vi "Software Initialisation.vi"(8 "error in (no error)":errorcluster, 11 "UI elements cluster":T2) -> (0 "Error Out":errorcluster, 2 "Event Registration Refnum":refnum<event-registration>, 3 "Message Queues out":T1)   [LabVIEW 2020]
uses:
  Typedefs/Top level VI states.ctl
  Typedefs/UI ctrl refs cluster.ctl
  Typedefs/Laser control knob.ctl
  Typedefs/Frame Size.ctl
  Typedefs/Plane Mode.ctl
  Typedefs/PMT control knob.ctl
  Typedefs/XY Stage_Move.ctl
  Typedefs/test_fpga_control.ctl
  Acquisition/Typedefs/Ref DAQ Param.ctl
  User Interface/Misc/Experiment Type.ctl
  User Interface/Misc/Biology Information.ctl
  User Interface/Queue/Message Queue/Typedefs/All Message Queues.ctl
  User Interface/Queue/Message Queue/Typedefs/Message Cluster.ctl
  Typedefs/Logging queue element.ctl
  Typedefs/Imaging Protocols enum.ctl
  Typedefs/Acquired points count.ctl
  Error window positioning/Error window pos FGV states.ctl
  Typedefs/Save-Load enum.ctl
  Global Variables/gl_UI Ctrl Refs.vi
  Global Variables/General Globals.vi
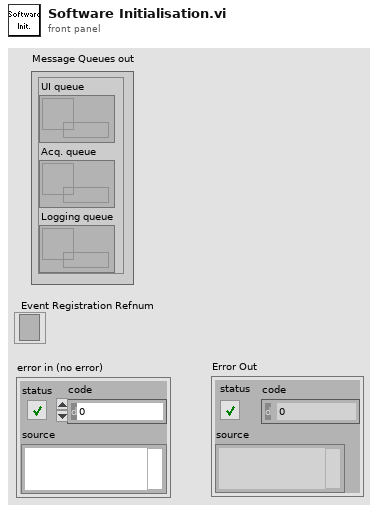
[diagram p1: front panel]
types:
  T1 = typedef "All Message Queues.ctl" = cluster{"UI queue":refnum<queue>, "Acq. queue":refnum<queue>, "Logging queue":refnum<queue>}
  T2 = typedef "UI ctrl refs cluster.ctl" = cluster{"Top level VI path":path, "Top level VI ref":refnum<vi>, "User menu ref":refnum<k9>, "Sub Panel control":refnum<vi>, "Imaging Param Tab":refnum<vi>, "Occurrence-Start drivers":refnum<k4>, "Occurrence-Speed logging initialised":refnum<k4>, "Occurrence-XYZ stage initialised":refnum<k4>, "Exit button":refnum<vi>, "Status ind":refnum<vi>, "Set as origin":refnum<vi>, "Speed Logging":refnum<vi>, "Time Lapse":refnum<vi>, "Live Imaging":refnum<vi>, "AOL Z Stack":refnum<vi>, "Motor Z Stack":refnum<vi>, "Funct Acq button":refnum<vi>, "Hard Shutter":refnum<vi>, "Virtual Shutter":refnum<vi>, "Laser Power":refnum<vi>, "AOL Mode":refnum<vi>, "Frame Size":refnum<vi>, "Field of View":refnum<vi>, "Dwell Time":refnum<vi>, "Zoom":refnum<vi>, "AOL Z":refnum<vi>, "Objective":refnum<vi>, "Axis":refnum<vi>, "Paths & Names":refnum<vi>, "Experiment folder path (ind.)":refnum<vi>, "Last State (Ind.)":refnum<vi>, "Averages":refnum<vi>, "Angle (degrees)":refnum<vi>, "X centre":refnum<vi>, "Y centre":refnum<vi>, "Plane Mode":refnum<vi>, "# Planes":refnum<vi>, "Z Start":refnum<vi>, "Z Stop":refnum<vi>, "Z Step":refnum<vi>, "PMT 1":refnum<vi>, "PMT 2":refnum<vi>, "Stage XYZ Position":refnum<vi>, "Pockels@Z Start":refnum<vi>, "Pockels@Z Stop":refnum<vi>, "Obtain Z Start":refnum<vi>, "Obtain Z Stop":refnum<vi>, "Live stim.trig.period":refnum<vi>, "Live stim.trig.enable":refnum<vi>, "Movement Correction":refnum<vi>, "Load Reference Image":refnum<vi>, "XY Stage Move":refnum<vi>, "MovCor Cluster":refnum<vi>, "RefDAQParam":refnum<vi>, "Funct. Acq. Pockels Modulation":refnum<vi>, "Ref Laser Power":refnum<vi>, "Enable Video Recording":refnum<vi>, "Video Record-Live Imaging":refnum<vi>, "Video Record-Funct acq":refnum<vi>, "Reference Source":refnum<vi>, "AOL Z-stack Chirps Ready (ind)":refnum<vi>, "Target time between mov.cor. ref triggers (ms)":refnum<vi>, "Funct. Acq. Ref frame save":refnum<vi>, "Tracking button":refnum<vi>, "Show ref plots window":refnum<vi>, "Center freq ind (nm)":refnum<vi>, "Pickup mode (ind)":refnum<vi>, "Logging queue (ind)":refnum<vi>, "Back aperture power (ind.)":refnum<vi>, "Power after objective (ind.)":refnum<vi>, "Switch user":refnum<vi>, "Ls1 Conn. Status":refnum<vi>, "Ls1Tuning Status":refnum<vi>, "Ls1 Faults":refnum<vi>, "Ls1 Connection":refnum<vi>, "Ls1 Mode":refnum<vi>, "Ls1 POWER [mW]":refnum<vi>, "Ls1Shutter":refnum<vi>, "Ls1 Wavelength":refnum<vi>, "Ls1 Note":refnum<vi>, "Ls1 Confirm Wav":refnum<vi>, "Ls1 PreChrp Prism1":refnum<vi>, "Ls1 PreChrp Prism2":refnum<vi>, "Ls1 wav top Ind":refnum<vi>, "Ls1 power top Ind":refnum<vi>, "Ls1 Pump peak Hold":refnum<vi>, "Ls1 Status Ind":refnum<vi>, "Ls1 wav cancel":refnum<vi>, "Experiment Type":refnum<vi>, "Biology Information":refnum<vi>, "Camera recording status":refnum<vi>, "Optimise Obj. Pos.":refnum<vi>}
  T3 = typedef "Save-Load enum.ctl" = enum16{"Save to file", "Load from file", "Compare from file", "Save Backup"}
  T4 = enum32{"Invalid", "Standard", "Closed", "Hidden", "Minimized", "Maximized"}
  T5 = typedef "Error window pos FGV states.ctl" = enum16{"Read", "Window closed", "Window opened", "Reset"}
  T6 = enum16{"Obtain queue", "Call window", "Call & send signal", "Release queue"}
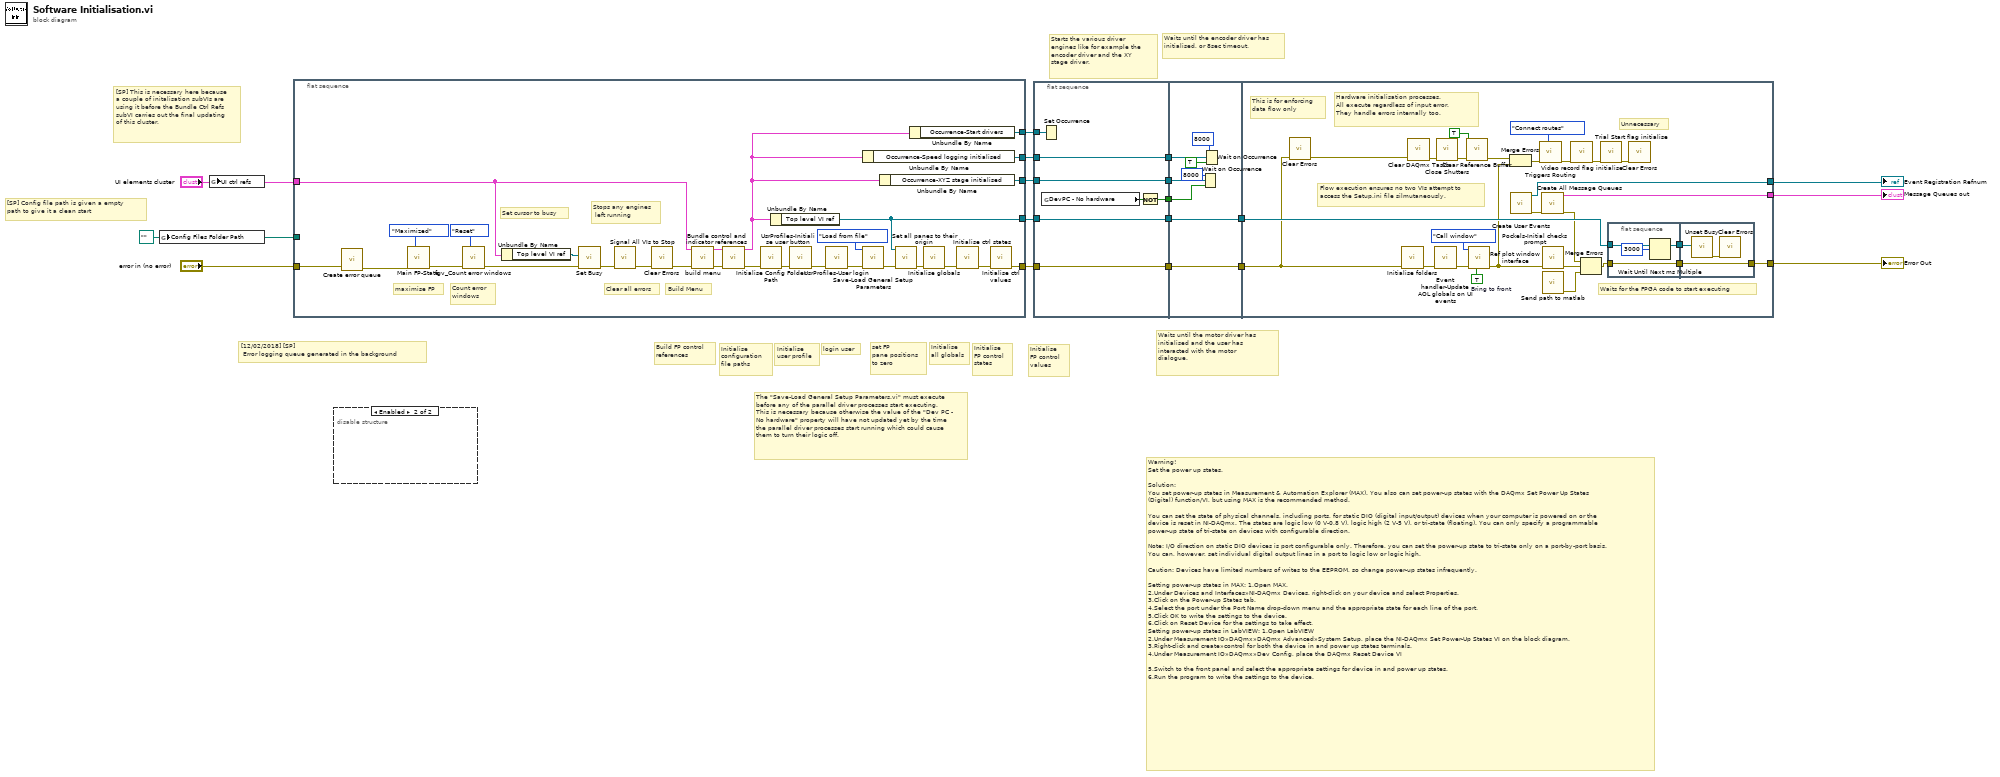
[diagram p0: block diagram]
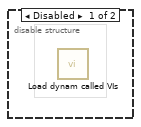
[diagram p2: hidden frame]
diagram:
  w13 = path "" ("Config Files Folder Path")
  # "[12/02/2018] [SP]\n Error logging queue generated in the background"
  # "[SP] Config file path is given a empty \npath to give it a clean start"
  # "Initialise \nFP control\nvalues"
  # "Initialise \nFP control\nstates"
  # "Initialise \nall globals"
  # "set FP \npane positions\nto zero"
  # "login user"
  # "Initialise \nuser profile"
  # "Initialise \nconfiguration\nfile paths"
  # "Build FP control\nreferences"
  # "Waits until the motor driver has initialised and the user has interacted with the motor dialogue."
  # "Starts the various driver engines like for example the encoder driver and the XY stage driver."
  # "Waits until the encoder driver has initialised, or 8sec timeout."
  # "The \"Save-Load General Setup Parameters.vi\" must execute before any of the parallel driver processes start executing. This is necessary because otherwise the value of the \"Dev PC - No hardware\" property will have not updated yet by the time the parallel driver processes start running which could cause them to turn their logic off."
  # "[SP] This is necessary here because a couple of initalisation subVIs are using it before the Bundle Ctrl Refs subVI carries out the final updating of this cluster."
  # "Warning!\nSet the power up states.\n\nSolution: \nYou set power-up states in Measurement & Automation Explorer (MAX). You also can set power-up states with the DAQmx Set Power Up States (Digital) function/VI, but using MAX is the recommended method. \n\nYou can set the state of physical channels, including ports, for static DIO (digital input/output) devices when your computer is powered on or the device is reset in NI-DAQmx. The states are logic low (0 V-0.8 V), logic high (2 V-5 V), or tri-state (floating). You can only specify a programmable power-up state of tri-state on devices with configurable direction. \n\nNote: I/O direction on static DIO devices is port configurable only. Therefore, you can set the power-up state to tri-state only on a port-by-port basis. You can, however, set individual digital output lines in a port to logic low or logic high.\n\nCaution: Devices have limited numbers of writes to the EEPROM, so change power-up states infrequently.\n\nSetting power-up states in MAX: 1.Open MAX.\n2.Under Devices and Interfaces»NI-DAQmx Devices, right-click on your device and select Properties.\n3.Click on the Power-up States tab.\n4.Select the port under the Port Name drop-down menu and the appropriate state for each line of the port.\n5.Click OK to write the settings to the device.\n6.Click on Reset Device for the settings to take effect.\nSetting power-up states in LabVIEW: 1.Open LabVIEW\n2.Under Measurement IO»DAQmx»DAQmx Advanced»System Setup, place the NI-DAQmx Set Power-Up States VI on the block diagram.\n3.Right-click and create»control for both the device in and power up states terminals.\n4.Under Measurement IO»DAQmx»Dev Config, place the DAQmx Reset Device VI \n\n5.Switch to the front panel and select the appropriate settings for device in and power up states.\n6.Run the program to write the settings to the device."
  n1 = global write "General Globals.vi" "Config Files Folder Path"(w13) -> ()
  n2 = global write "gl_UI Ctrl Refs.vi" "UI ctrl refs"("UI elements cluster") -> ()
  n3 = flat-sequence {
    tunnel: "error in (no error)" -> [w21]
    tunnel: "UI elements cluster" -> [w38]
    tunnel: [w34] -> w8
    tunnel: [w33] -> w9
    tunnel: [w32] -> w10
    tunnel: [w31] -> w11
    tunnel: w13 -> [_]
    tunnel: [w30] -> w12
    frame #0 {
      # "Build Menu"
      # "Clear all errors"
      # "Stops any engines\n left running"
      # "Set cursor to busy"
      # "maximise FP"
      # "Count error\nwindows"
      n4 = call "Create error queue.vi"("Error in"=w21) -> ("Error out"=w20:errorcluster)  [unwired: 10 in]
      n5 = call "Main FP-State.vi"("error in (no error)"=w20, "Front Panel Window:State"=T4."Maximized") -> ("error out"=w39:errorcluster)  [unwired: 9 in]
      n6 = call "fgv_Count error windows.vi"("error in (no error)"=w39, "Function"=Error_window_pos_FGV_states."Reset") -> ("error out"=w41:errorcluster)  [unwired: 7 in, 2 out]
      n7 = Unbundle By Name(w38) -> ("Top level VI ref"=w44:refnum<vi>)
      n8 = call <vilib>:"Set Busy.vi"("error in (no error)"=w41, "VI reference (current VI)"=w44) -> ("error out"=w46:errorcluster)  [unwired: 8 in, 1 out]
      n9 = call "Signal All VIs to Stop.vi"("error in (no error)"=w46) -> ("error out"=w36:errorcluster)  [unwired: 10 in]
      n10 = call <vilib>:"Clear Errors.vi"("error in (no error)"=w36) -> ("error out"=w35:errorcluster)  [unwired: 5 in, 1 out]
      n11 = call "build menu.vi"("error in (no error)"=w35, "UI elements cluster"=w38) -> ("error out"=w45:errorcluster, "UI elements cluster"=w37:T2)  [unwired: 8 in]
      n12 = call "Bundle control and indicator references.vi"("error in"=w45, "UI elements cluster"=w37) -> ("error out"=w19:errorcluster, "UI elements cluster"=w29:T2)  [unwired: 8 in]
      n13 = call "Initialise Config Folder Path.vi"("error in (no error)"=w19) -> ("error out"=w43:errorcluster)  [unwired: 8 in, 2 out]
      n14 = Unbundle By Name(w29) -> ("Top level VI ref"=w31:refnum<vi>)
      n15 = call "UsrProfiles-Initialise user button.vi"("error in (no error)"=w43) -> ("error out"=w28:errorcluster)  [unwired: 10 in]
      n16 = call "UsrProfiles-User login.vi"("error in (no error)"=w28) -> ("error out"=w26:errorcluster)  [unwired: 10 in]
      n17 = Unbundle By Name(w29) -> ("Occurrence-Speed logging initialised"=w33:refnum<k4>)
      n18 = call "Save-Load General Setup Parameters.vi"("error in"=w26, "Function"=Save-Load_enum."Load from file") -> ("error out"=w23:errorcluster)  [unwired: 9 in]
      n19 = Unbundle By Name(w29) -> ("Occurrence-XYZ stage initialised"=w32:refnum<k4>)
      n20 = call <userlib>:"Set all panes to their origin.vi"("error in (no error)"=w23, "Top level VI ref"=w31) -> ("error out"=w22:errorcluster)  [unwired: 9 in]
      n21 = Unbundle By Name(w29) -> ("Occurrence-Start drivers"=w34:refnum<k4>)
      n22 = call "Initialise globals.vi"("error in (no error)"=w22) -> ("error out"=w25:errorcluster)  [unwired: 10 in]
      n23 = call "Initialise ctrl states.vi"("error in (no error)"=w25) -> ("error out"=w24:errorcluster)  [unwired: 10 in]
      n24 = call "Initialise ctrl values.vi"("error in (no error)"=w24) -> ("error out"=w30:errorcluster)  [unwired: 10 in]
    }
  }
  n25 = disable-structure shown="Enabled" {
    frame Disabled {
      n26 = call "Load dynam called VIs.vi"() -> ()  [unwired: 12 in]
    }
    frame Enabled {
    }
  }
  n27 = flat-sequence {
    tunnel: [w48] -> w7
    tunnel: [w49] -> w6
    tunnel: [w51] -> w5
    tunnel: [w50] -> w4
    tunnel: [w52] -> w3
    tunnel: w12 -> [w51]
    tunnel: w11 -> [w50]
    tunnel: w10 -> [w49]
    tunnel: w9 -> [w48]
    tunnel: w8 -> [w47]
    tunnel: [w58] -> w2
    tunnel: w7 -> [w61]
    tunnel: w6 -> [w60]
    tunnel: w5 -> [w58]
    tunnel: [w57] -> w1
    tunnel: w4 -> [w57]
    tunnel: w3 -> [w55]
    tunnel: [w88] -> w18
    tunnel: w2 -> [w64]
    tunnel: [w87] -> w17
    tunnel: [w86] -> w16
    tunnel: w1 -> [w85]
    frame #0 {
      n28 = Set Occurrence(w47) -> ()
      n29 = global read "General Globals.vi" "DevPC - No hardware"() -> (w53:bool)
      n30 = Not(x=w53) -> (.not. x?=w52:bool)
    }
    frame #1 {
      n31 = Wait on Occurrence(1:w55, 2:w60, 3:8000 ("ms timeout (-1)")) -> ()  [unwired: 1 out]
      n32 = Wait on Occurrence(1:TRUE ("ignore previous (T)"), 2:w61, 3:8000 ("ms timeout (-1)")) -> ()  [unwired: 1 out]
    }
    frame #2 {
      w76 = TRUE  # Bring to front
      # "This is for enforcing\ndata flow only"
      # "Hardware initialisation processes. \nAll execute regardless of input error.\nThey handle errors internally too."
      # "Unnecessary"
      # "Waits for the FPGA code to start executing"
      # "Flow execution ensures no two VIs attempt to access the Setup.ini file silmutaneously."
      n33 = call <vilib>:"Clear Errors.vi"("error in (no error)"=w64) -> ("error out"=w63:errorcluster)  [unwired: 5 in, 1 out]
      n34 = call "Initialise folders.vi"("error in (no error)"=w64) -> ("error out"=w81:errorcluster)  [unwired: 10 in]
      n35 = call "Clear DAQmx Tasks.vi"("error in (no error)"=w63) -> ("error out"=w65:errorcluster)  [unwired: 10 in]
      n36 = call "Event handler-Update AOL globals on UI events.vi"("error in (no error)"=w81) -> ("error out"=w77:errorcluster)  [unwired: 10 in]
      n37 = call "Close Shutters.vi"("error in (no error)"=w65) -> ("error out (no error)"=w70:errorcluster)  [unwired: 10 in]
      n38 = call "Clear Reference Buffer.vi"("error in (no error)"=w70, "Ethernet port opened"=TRUE) -> ("error out"=w66:errorcluster)  [unwired: 9 in]
      n39 = call "Ref plot window interface.vi"("Bring to front (F)"=w76, "error in (no error)"=w77, "Function"=T6."Call window") -> ("error out"=w73:errorcluster)  [unwired: 7 in, 1 out]
      n40 = Merge Errors(w66, w73) -> (w67:errorcluster)
      n41 = call "Create User Events.vi"() -> ("Error Out"=w82:errorcluster, "Event Registration Refnum"=w88:refnum<event-registration>)  [unwired: 10 in]
      n42 = call "Triggers Routing.vi"("Function"=enum16{"Connect routes", "Disconnect routes"}."Connect routes", "error in (no error)"=w67) -> ("error out (no error)"=w71:errorcluster)  [unwired: 9 in]
      n43 = call "Create All Message Queues.vi"("Error In"=w82) -> ("Error Out"=w80:errorcluster, "Message Queues out"=w86:T1)  [unwired: 9 in]
      n44 = call "Pockels-Initial checks prompt.vi"("error in (no error)"=w73) -> ("error out"=w75:errorcluster)  [unwired: 10 in]
      n45 = call "Send path to matlab.vi"() -> ("error out"=w74:errorcluster)  [unwired: 11 in]
      n46 = call "Video record flag initialise.vi"("error in (no error)"=w71) -> ("error out (no error)"=w72:errorcluster)  [unwired: 10 in]
      n47 = Merge Errors(w80, w75, w74) -> (w79:errorcluster)
      n48 = call "Trial Start flag initialise.vi"("error in (no error)"=w72) -> ("error out (no error)"=w68:errorcluster)  [unwired: 10 in]
      n49 = flat-sequence {
        tunnel: w85 -> [w91]
        tunnel: [w91] -> w84
        tunnel: w79 -> [w89]
        tunnel: [w89] -> w83
        tunnel: w84 -> [w94]
        tunnel: w83 -> [w92]
        tunnel: [w92] -> w87
        frame #0 {
          n50 = Wait Until Next ms Multiple(millisecond multiple=u32 3000) -> ()  [unwired: 1 out]
        }
        frame #1 {
          n51 = call <vilib>:"Unset Busy.vi"("VI reference (current VI)"=w94) -> ("error out"=w93:errorcluster)  [unwired: 10 in]
          n52 = call <vilib>:"Clear Errors.vi"("error in (no error)"=w93) -> ()  [unwired: 5 in, 2 out]
        }
      }
      n53 = call <vilib>:"Clear Errors.vi"("error in (no error)"=w68) -> ()  [unwired: 5 in, 2 out]
    }
  }
  "Error Out" <- w17
  "Event Registration Refnum" <- w18
  "Message Queues out" <- w16
